vi "Parse String.vi"(7 "conversion blocks":T1[](array[typedef]) {"string offset" format="%d bytes"; "engine offset" format="%d bytes"}, 8 "error in (no error)":errorcluster, 10 "engine buffer in":u8[](array[numeric]), 11 "string buffer in":u8[](array[numeric])) -> (0 "error out":errorcluster, 2 "engine buffer out":u8[](array[numeric]), 3 "string buffer out":u8[](array[numeric]))   [LabVIEW 2017, in "DSF Core.lvlib" / "DSF Buffer Converter.lvclass"]
uses:
  DSF Buffer Converter.lvclass
  Conversion Block.ctl
  Typedefs/DSF Data Type.ctl
  VIs/Sizeof 1D.vi
  DSF Core.lvlib
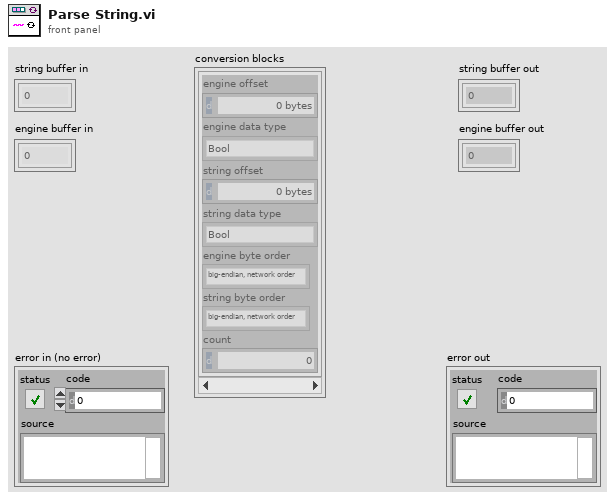
[diagram p1: front panel]
types:
  T1 = typedef "DSF Core.lvlib/DSF Buffer Converter.lvclass/Conversion Block.ctl" = cluster{"engine offset":u64, "engine data type":T2, "string offset":u64, "string data type":T2, "engine byte order":enum16{"big-endian, network order", "native, host order", "little-endian"}, "string byte order":enum16{"big-endian, network order", "native, host order", "little-endian"}, "count":u64}
  T2 = typedef "DSF Core.lvlib/DSF Data Type.ctl" = enum8{"Bool", "SGL", "DBL", "I8", "I16", "I32", "I64", "U8", "U16", "U32", "U64"}
  T3 = enum16{"big-endian, network order", "native, host order", "little-endian"}
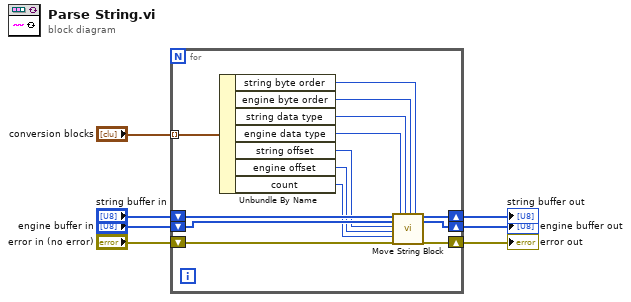
[diagram p0: block diagram]
diagram:
  n1 = for {
    tunnel: "conversion blocks" -> [w20] mode=indexing
    shift-right: [w19] -> w3
    shift-left: "error in (no error)" -> [w21]
    shift-right: [w18] -> w7
    shift-left: "engine buffer in" -> [w16]
    shift-right: [w17] -> w6
    shift-left: "string buffer in" -> [w15]
    n2 = Unbundle By Name(w20) -> ("string byte order"=w8:T3, "engine byte order"=w9:T3, "string data type"=w10:T2, "engine data type"=w11:T2, "string offset"=w12:u64, "engine offset"=w13:u64, "count"=w14:u64)
    n3 = call "Move String Block.vi"("src buffer in"=w15, "dst buffer in"=w16, "src buffer offset"=w12, "dst buffer offset"=w13, "channel count"=w14, "error in (no error)"=w21, "dst data type"=w11, "src data type"=w10, "dst byte order"=w9, "src byte order"=w8) -> ("src buffer out"=w17:u8[], "dst buffer out"=w18:u8[], "error out"=w19:errorcluster)  [unwired: 7 in]
  }
  "string buffer out" <- w6
  "engine buffer out" <- w7
  "error out" <- w3
